vi "SectionA04_Week7_Stus.vi"() -> ()   [LabVIEW 2013]
panel:
  in  "?":bool
  in  "Y":dbl(knob) scale=0.0..10.0
  in  "X":dbl(knob) scale=0.0..10.0
  out "Etch-a-Sketch":cluster{dbl[], dbl[]}(graph)
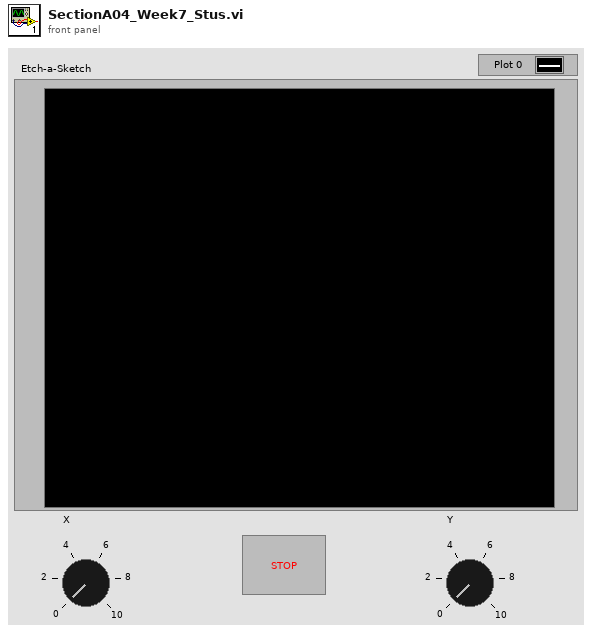
[diagram p1: front panel]
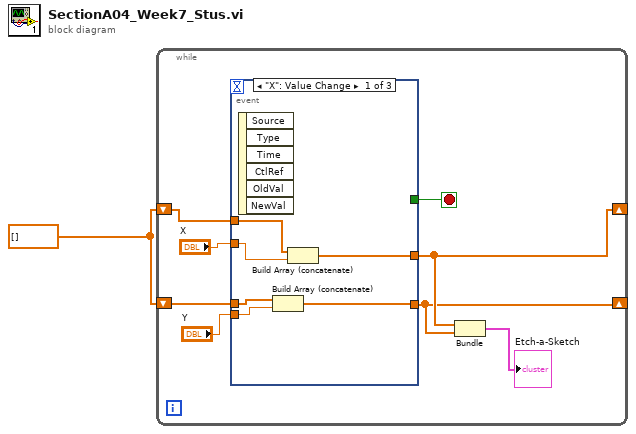
[diagram p0: block diagram]
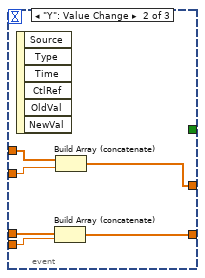
[diagram p2: hidden frame]
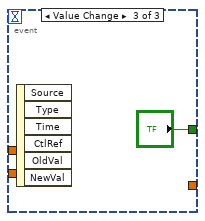
[diagram p3: hidden frame]
diagram:
  w1 = dbl[] []
  n1 = while {
    shift-right: [w4] -> _
    shift-left: w1 -> [w6]
    shift-right: [w3] -> _
    shift-left: w1 -> [w5]
    stop <- w9 stop-if-true
    n2 = event "\"stop\"" shown="[0] \"X\": Value Change" {
      selector: _ -> [_ _ _]
      dyn-events: _ -> [_ _ _]
      timeout: _ -> [_ _ _]
      tunnel: [_ _ "?"] -> w9
      tunnel: "X" -> [w14 w17 _]
      tunnel: "Y" -> [w11 w20 _]
      tunnel: w6 -> [w15 w18 _]
      tunnel: w5 -> [w12 w21 _]
      tunnel: [w13 w16 _] -> w4
      tunnel: [w10 w19 _] -> w3
      event "X": Value Change {
        n3 = event-data() -> ()  [unwired: 1 in, 6 out]
        n4 = Build Array (concatenate)(w12, w11) -> (w10:dbl[])
        n5 = Build Array (concatenate)(w15, w14) -> (w13:dbl[])
      }
      event "Y": Value Change {
        n6 = event-data() -> ()  [unwired: 1 in, 6 out]
        n7 = Build Array (concatenate)(w21, w20) -> (w19:dbl[])
        n8 = Build Array (concatenate)(w18, w17) -> (w16:dbl[])
      }
      event Value Change {
        n9 = event-data() -> ()  [unwired: 1 in, 6 out]
      }
    }
    n10 = Bundle(w4, w3) -> (→"Etch-a-Sketch":cluster{dbl[], dbl[]})  [unwired: 1 in]
  }
